vi "PIDantiWindup.vi"(8 "PID Gains":cluster{"Kp":dbl, "Kd":dbl, "Ki":dbl}, 9 "Saturation":dbl[](array[numeric]), 10 "Position":dbl, 11 "Reference":dbl) -> (3 "control":dbl)   [LabVIEW 2018, in "kevLib2011.lvlib"]
uses:
  kevLib2011.lvlib
panel:
  # "Not Tested Yet"
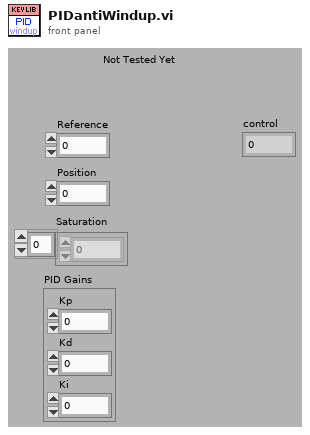
[diagram p1: front panel]
types:
  T1 = cluster{"[0]":dbl, "[1]":dbl, "[2]":dbl, "[3]":dbl, "[4]":dbl, "[5]":dbl, "[6]":dbl, "[7]":dbl, "[8]":dbl}
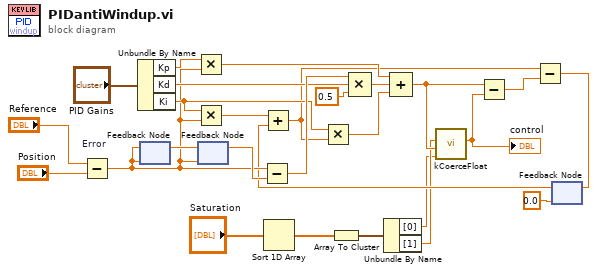
[diagram p0: block diagram]
diagram:
  n1 = Subtract "Error"(x="Reference", y="Position") -> (x-y=w13:dbl)
  n2 = Unbundle By Name("PID Gains") -> ("Kp"=w24:dbl, "Kd"=w19:dbl, "Ki"=w14:dbl)
  n3 = feedback-in #1(w13) -> ()
  n4 = feedback #1(w13) -> (w22:dbl)
  n5 = Multiply(x=w24, y=w13) -> (x*y=w23:dbl)
  n6 = Multiply(x=w14, y=w13) -> (x*y=w12:dbl)
  n7 = feedback-in #2(w22) -> ()
  n8 = feedback #2(w13) -> (w21:dbl)
  n9 = Subtract(x=w13, y=w21) -> (x-y=w20:dbl)
  n10 = Sort 1D Array(array="Saturation") -> (sorted array=w4:dbl[])
  n11 = Array To Cluster(array=w4) -> (cluster=w3:T1)
  n12 = Compound Arithmetic op=MULTIPLY(w20, w19, 0.5 ("value")) -> (w17:dbl)
  n13 = Unbundle By Name(w3) -> ("[0]"=w1:dbl, "[1]"=w2:dbl)
  n14 = feedback #3(0.0 ("value")) -> (w11:dbl)
  n15 = Add(x=w12, y=w11) -> (x+y=w7:dbl)
  n16 = Multiply(x=w14, y=w7) -> (x*y=w15:dbl)
  n17 = Compound Arithmetic op=ADD(w23, w17, w15) -> (w10:dbl)
  n18 = call "kCoerceFloat.vi"("lower"=w1, "input"=w10, "upper"=w2) -> ("output"=w9:dbl)  [unwired: 7 in, 1 out]
  "control" <- w9
  n19 = Subtract(x=w10, y=w9) -> (x-y=w8:dbl)
  n20 = Subtract(x=w7, y=w8) -> (x-y=w6:dbl)
  n21 = feedback-in #3(w6) -> ()
